vi "Read Housing Size.vi"(9 "NumericWithScale in":refnum<class "NumericWithScale.lvclass">) -> (3 "NumericWithScale out":refnum<class "NumericWithScale.lvclass">, 4 "Housing Size":T1)   [LabVIEW 2014, in "NumericWithScale.lvclass"]
uses:
  NumericWithScale.lvclass
  <vilib>/Utility/miscctls.llb/LVBoundsTypeDef.ctl
  NumericWithScale.lvclass/NumericWithScale.ctl
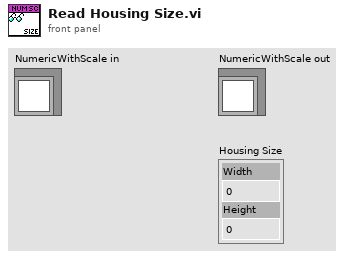
[diagram p1: front panel]
types:
  T1 = typedef "LVBoundsTypeDef.ctl" = cluster{"Width":u32, "Height":u32}
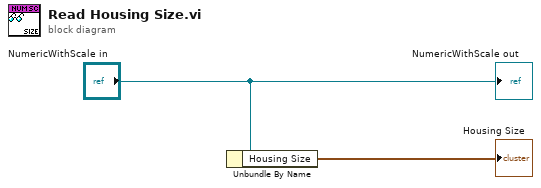
[diagram p0: block diagram]
diagram:
  n1 = Unbundle By Name("NumericWithScale in") -> ("Housing Size"=→"Housing Size":T1)
  "NumericWithScale out" <- "NumericWithScale in"
